vi "FTW-Listener-Construct.vi"(0 "FTW-Listener-LVQ In":refnum<class "FTW-Listener-LVQ.lvclass">, 5 "Address":string, 11 "error in":errorcluster) -> (4 "FTW-Listener-LVQ Out":refnum<class "FTW-Listener-LVQ.lvclass">, 15 "error out":errorcluster)   [LabVIEW 2013, in "FTW-Listener-LVQ.lvclass"]
uses:
  FTW-Listener-LVQ.lvclass
  Listener/FTW-Listener.lvclass
  FTW-Listener-LVQ.lvclass/FTW-Listener-LVQ.ctl
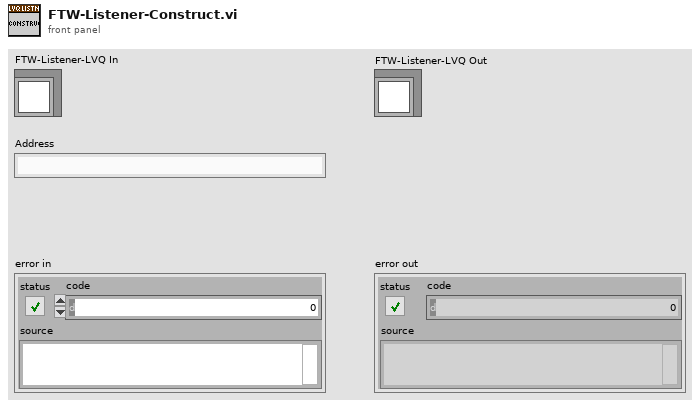
[diagram p1: front panel]
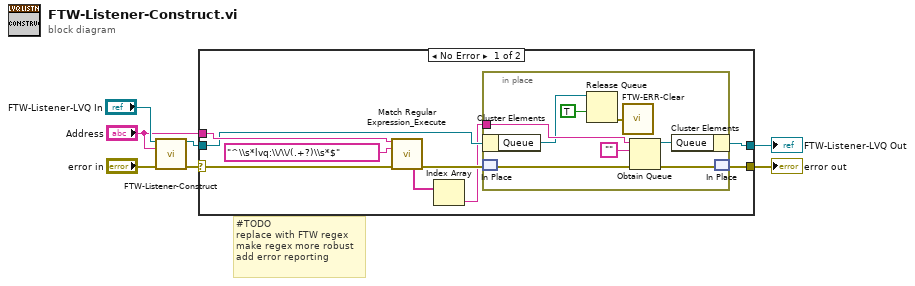
[diagram p0: block diagram]
diagram:
  # "#TODO\nreplace with FTW regex\nmake regex more robust\nadd error reporting"
  n1 = call-parent "FTW-Listener-Construct.vi"("Gmsg_Listener In"="FTW-Listener-LVQ In", "Address"="Address", "error in"="error in") -> ("Gmsg_Listener Out"=w2:refnum<class "FTW-Listener-LVQ.lvclass">, "error out"=w4:errorcluster)  [unwired: 11 in]
  n2 = case shown="No Error" w4 {
    selector: w4 -> [w12 w26]
    tunnel: [w16 w26] -> w6
    tunnel: [w15 w25] -> w5
    tunnel: "Address" -> [w13 _]
    tunnel: w2 -> [w9 w25]
    frame No Error {
      n3 = call <vilib>:"Match Regular Expression_Execute.vi"("input string"=w13, "regular expression"="^\\s*lvq:\\/\\/(.+?)\\s*$" ("input string"), "error in (no error)"=w12) -> ("matched substrings"=w10:string[], "error out"=w11:errorcluster)  [unwired: 7 in, 4 out]
      n4 = Index Array(array=w10) -> (element=w8:string)  [unwired: 1 in]
      n5 = in-place {
        in-place-border: w8 -> [w21]
        n6 = in-place-cluster #1(w9) -> ("Queue"=w19:refnum<queue>)
        n7 = in-place-match #2(w11) -> (w24:errorcluster)
        n8 = Release Queue(queue=w19, force destroy? (F)=TRUE) -> (error out=w17:errorcluster)  [unwired: 1 in, 2 out]
        n9 = call "FTW-ERR-Clear.vi"("error to snuff"=w17) -> ()  [unwired: 1 out]
        n10 = Obtain Queue(name (unnamed)=w21, element data type="", error in (no error)=w24) -> (queue out=w22:refnum<queue>, error out=w23:errorcluster)  [unwired: 2 in, 1 out]
        n11 = in-place-cluster #1("Queue"=w22) -> (w15:refnum<class "FTW-Listener-LVQ.lvclass">)
        n12 = in-place-match #2(w23) -> (w16:errorcluster)
      }
    }
    frame Error {
    }
  }
  "FTW-Listener-LVQ Out" <- w5
  "error out" <- w6
